vi "the_greatest.vi"(2 "A":dbl, 3 "B":dbl) -> (7 "Greatest":dbl)   [LabVIEW 2015]
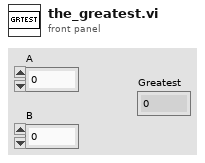
[diagram p1: front panel]
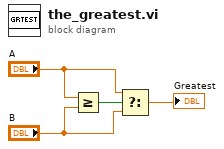
[diagram p0: block diagram]
diagram:
  n1 = Greater Or Equal?(x="A", y="B") -> (x >= y?=w1:bool)
  n2 = Select(t="A", s=w1, f="B") -> (s? t:f=→"Greatest":dbl)
